vi "v0.2_pto_serial.vi"(8 "error in (no error)":errorcluster, 10 "Fout":u32, 11 "VISA COM IN":refnum<visa-resource-name>) -> (0 "error out":errorcluster, 3 "VISA COM OUT":refnum<visa-resource-name>)   [LabVIEW 2011]
doc: "<B>PTO Salida de tren de pulsos</B>\n\nCambiar la frecuencia de salida. Un valor de cero detiene el motor. Existe un valor máximo luego del cual el servomotor se detiene, este valor depende de los paràmetros del driver.\n<B>Frecuencia </B> Valor en hertzios del tren de pulsos a la salida del microcontrolador mbed."
panel:
  # "Cambiar la frecuencia de salida"
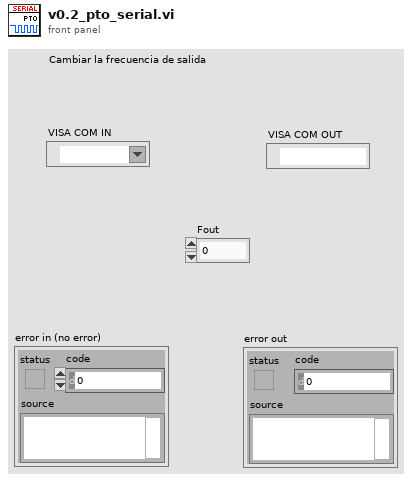
[diagram p1: front panel]
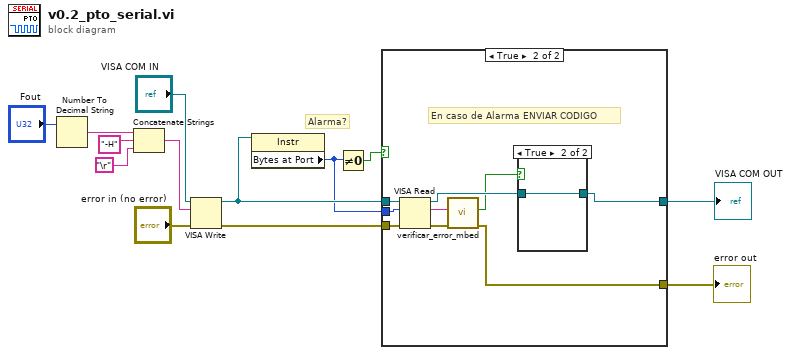
[diagram p0: block diagram]
diagram:
  # "Alarma?"
  n1 = Number To Decimal String(number="Fout") -> (decimal integer string=w13:string)  [unwired: 1 in]
  n2 = Concatenate Strings(w13, "-H" ("string"), "\r") -> (w11:string)
  n3 = VISA Write(VISA resource name="VISA COM IN", write buffer=w11, error in (no error)="error in (no error)") -> (VISA resource name out=w5:refnum<visa-resource-name>, error out=w7:errorcluster)  [unwired: 1 out]
  n4 = property class="Instr"(reference=w5) -> ("Bytes at Port"=w3:u32)  [unwired: 1 in, 2 out]
  n5 = Not Equal To 0?(x=w3) -> (x != 0?=w4:bool)
  n6 = case shown="True" w4 {
    tunnel: w5 -> [w15 w21]
    tunnel: w7 -> [w14 w20]
    tunnel: w3 -> [_ w18]
    tunnel: [w15 w17] -> w2
    tunnel: [w14 w16] -> w1
    frame False {
    }
    frame True {
      # "En caso de Alarma ENVIAR CODIGO"
      n7 = VISA Read(VISA resource name=w21, byte count=w18, error in (no error)=w20) -> (VISA resource name out=w22:refnum<visa-resource-name>, read buffer=w23:string, error out=w24:errorcluster)  [unwired: 1 out]
      n8 = call "verificar_error_mbed.vi"("error in (no error)"=w24, "desde_mbed"=w23) -> ("error out"=w16:errorcluster, "error?"=w19:bool)  [unwired: 8 in]
      n9 = case shown="True" w19 {
        tunnel: w22 -> [w25 w26]
        tunnel: [w25 w26] -> w17
        frame False {
        }
        frame True {
        }
      }
    }
  }
  "VISA COM OUT" <- w2
  "error out" <- w1
